vi "Configure IQ Recorder Measurement Trigger Phase Change.vi"(7 "Time (10.0e-6)":dbl=1e-05 format="%^.3e", 8 "error in (no error)":errorcluster, 9 "Threshold (45)":i32=45, 10 "Instance (1)":i32=1, 11 "VISA resource name":refnum<visa-resource-name>) -> (0 "error out":errorcluster, 3 "VISA resource name out":refnum<visa-resource-name>)   [LabVIEW 2020, in "Rohde&Schwarz CMXP GPRF.lvlib"]
doc: "This VI configures the trigger phase change. \n\nAttribute(s):\nRSCMXPGPRF_ATTR_IQ_RECORDER_MEASUREMENT_TRIGGER_PHASE_CHANGE_THRESHOLD\nRSCMXPGPRF_ATTR_IQ_RECORDER_MEASUREMENT_TRIGGER_PHASE_CHANGE_TIME\n\nRemote-control command(s):\nTRIGger:GPRF:MEAS<i>:IQRecorder:PCTHreshold\nTRIGger:GPRF:MEAS<i>:IQRecorder:PCTime"
uses:
  <instrlib>/Rohde&Schwarz CMXP GPRF/Rohde&Schwarz CMXP GPRF.lvlib
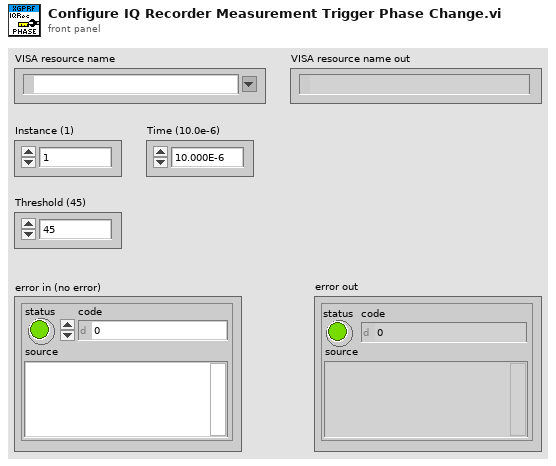
[diagram p1: front panel]
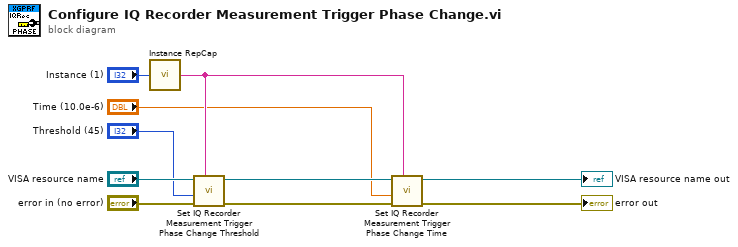
[diagram p0: block diagram]
diagram:
  n1 = call <instrlib>:"Instance RepCap.vi"("Instance in"="Instance (1)") -> ("Instance out"=w4:string)
  n2 = call "Set IQ Recorder Measurement Trigger Phase Change Threshold"("Repeated Capabilities"=w4, "error in (no error)"="error in (no error)", "IQ Recorder Measurement Trigger Phase Change Threshold (0)"="Threshold (45)", "instrument handle"="VISA resource name") -> ("error out"=w5:errorcluster, "instrument handle out"=w6:refnum<visa-resource-name>)  [unwired: 6 in]
  n3 = call "Set IQ Recorder Measurement Trigger Phase Change Time"("Repeated Capabilities"=w4, "error in (no error)"=w5, "IQ Recorder Measurement Trigger Phase Change Time (0.0)"="Time (10.0e-6)", "instrument handle"=w6) -> ("error out"=→"error out":errorcluster, "instrument handle out"=→"VISA resource name out":refnum<visa-resource-name>)  [unwired: 6 in]
